vi "TestStuff.vi"() -> ()   [LabVIEW 2022 SP3]
panel:
  in  "Map":map{dbl, string}(c390)
  out "x = y?":bool
  in  "Pswd":string
  in  "Usr":string
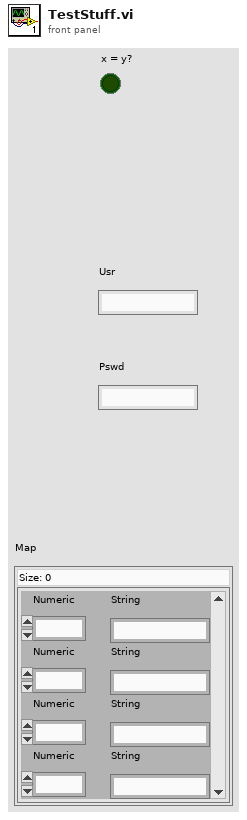
[diagram p1: front panel]
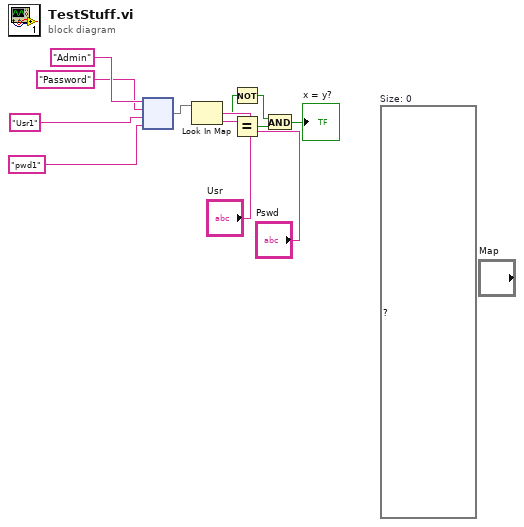
[diagram p0: block diagram]
diagram:
  (unwired) map{string, i32} {}  # Size: 0
  n1 = node("Admin", "Password", "Usr1", "pwd1") -> (w10:map{string, string})
  n2 = Look In Map(map=w10, key="Usr") -> (key not found?=w6:bool, value=w7:string)  [unwired: 1 in]
  n3 = Not(x=w6) -> (.not. x?=w5:bool)
  n4 = Equal?(x=w7, y="Pswd") -> (x = y?=w4:bool)
  n5 = And(x=w5, y=w4) -> (x .and. y?=→"x = y?":bool)
